vi "回文数质数算法1.vi"(3 "上限":dbl) -> (0 "回文质数数量":dbl, 1 "回文质数":dbl[](array[numeric]))   [LabVIEW 2017]
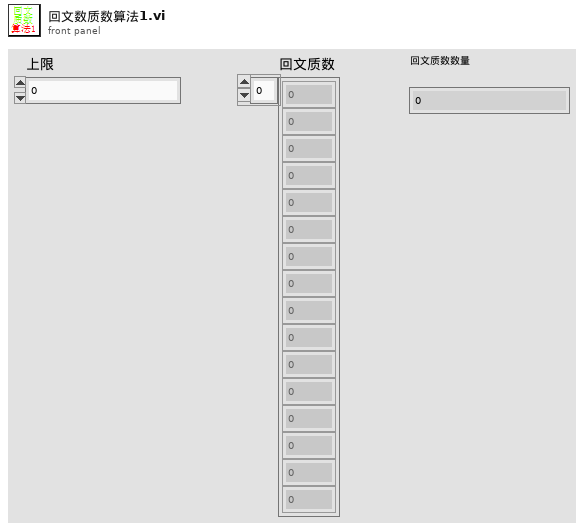
[diagram p1: front panel]
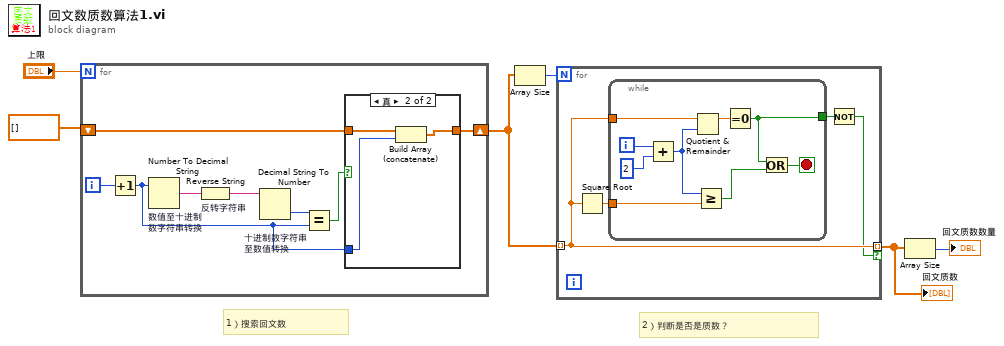
[diagram p0: block diagram]
diagram:
  # "2）判断是否是质数？"
  # "1）搜索回文数"
  n1 = for {
    N: "上限" -> [_]
    shift-right: [w9] -> w4
    shift-left: dbl[] [] -> [w10]
    i -> [w11]
    n2 = Increment(x=w11) -> (x+1=w7:i32)
    n3 = Number To Decimal String "数值至十进制\n数字符串转换"(number=w7) -> (decimal integer string=w13:string)  [unwired: 1 in]
    n4 = Reverse String "反转字符串"(1:w13) -> (0:w14:string)
    n5 = Decimal String To Number "十进制数字符串\n至数值转换"(string=w14) -> (number=w12:i32)  [unwired: 2 in, 1 out]
    n6 = Equal?(x=w12, y=w7) -> (x = y?=w8:bool)
    n7 = case shown="真" w8 {
      tunnel: w10 -> [w15 w18]
      tunnel: [w15 w17] -> w9
      tunnel: w7 -> [_ w16]
      frame False {
      }
      frame True {
        n8 = Build Array (concatenate)(w18, w16) -> (w17:dbl[])
      }
    }
  }
  n9 = Array Size(array=w4) -> (size(s)=w6:i32)
  n10 = for {
    N: w6 -> [_]
    tunnel: w4 -> [w20] mode=indexing
    tunnel: [w20] -> w1 mode=indexing if=w19
    n11 = Square Root(x=w20) -> (sqrt(x)=w22:dbl)
    n12 = while {
      tunnel: w22 -> [w27]
      tunnel: [w23] -> w21
      tunnel: w20 -> [w24]
      i -> [w30]
      stop <- w31 stop-if-true
      n13 = Add(x=w30, y=2) -> (x+y=w25:i32)
      n14 = Quotient & Remainder(x=w24, y=w25) -> (x-y*floor(x/y)=w28:dbl)  [unwired: 1 out]
      n15 = Greater Or Equal?(x=w25, y=w27) -> (x >= y?=w26:bool)
      n16 = Equal To 0?(x=w28) -> (x = 0?=w23:bool)
      n17 = Or(x=w23, y=w26) -> (x .or. y?=w31:bool)
    }
    n18 = Not(x=w21) -> (.not. x?=w19:bool)
  }
  "回文质数" <- w1
  n19 = Array Size(array=w1) -> (size(s)=→"回文质数数量":i32)
